vi "Read PAR_names.vi"(8 "error in (no error)":errorcluster, 11 "Param in":T1) -> (0 "error out":errorcluster, 2 "PAR_names":string[][](array[string]), 3 "Param out":T1)   [LabVIEW 2019, in "Inputs.lvlib"]
uses:
  Inputs.lvlib
  Ctl/Param.ctl
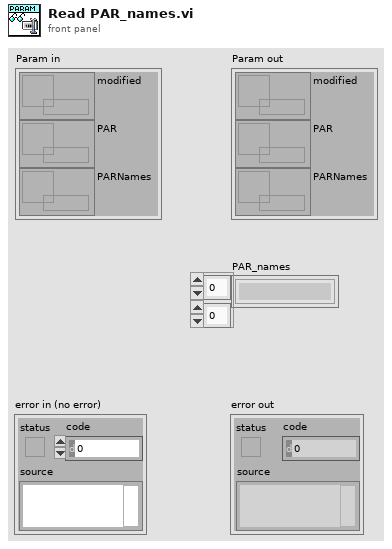
[diagram p1: front panel]
types:
  T1 = typedef "Inputs.lvlib/Param.ctl" = cluster{"modified":refnum<data-value>, "PAR":refnum<data-value>, "PARNames":refnum<data-value>}
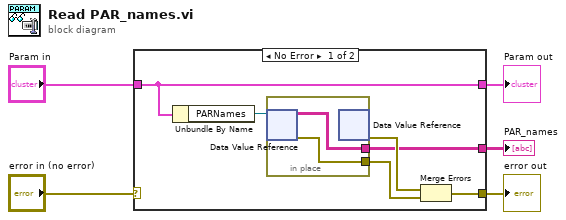
[diagram p0: block diagram]
diagram:
  n1 = case shown="No Error" "error in (no error)" {
    selector: "error in (no error)" -> [_ w14]
    tunnel: [w6 w14] -> w4
    tunnel: [w8 w15] -> w2
    tunnel: "Param in" -> [w8 w15]
    tunnel: [w7 _] -> w1
    frame No Error {
      n2 = Unbundle By Name(w8) -> ("PARNames"=w11:refnum<data-value>)
      n3 = in-place {
        in-place-border: [w13] -> w10
        in-place-border: [w12] -> w7
        n4 = in-place-dvr #1(w11) -> (w12:string[][], w13:errorcluster)
        n5 = in-place-dvr #1() -> (w9:errorcluster)  [unwired: 1 in, 1 out]
      }
      n6 = Merge Errors(w9, w10) -> (w6:errorcluster)
    }
    frame Error {
    }
  }
  "error out" <- w4
  "Param out" <- w2
  "PAR_names" <- w1
